vi "CRYFlatten User Equation Cluster.vi"(11 "user equation cluster":T1 {"Results axis" items=["x", "y", "z"]; "Input axis" items=["x", "y", "z"]; "Custom unit results array"."dB ref" format="%.2f"; "Custom unit input array"."dB ref" format="%.2f"}) -> (3 "Flatten String":string)   [LabVIEW 2013]
uses:
  Typedef Control/CRYUser Equation Cluster.ctl
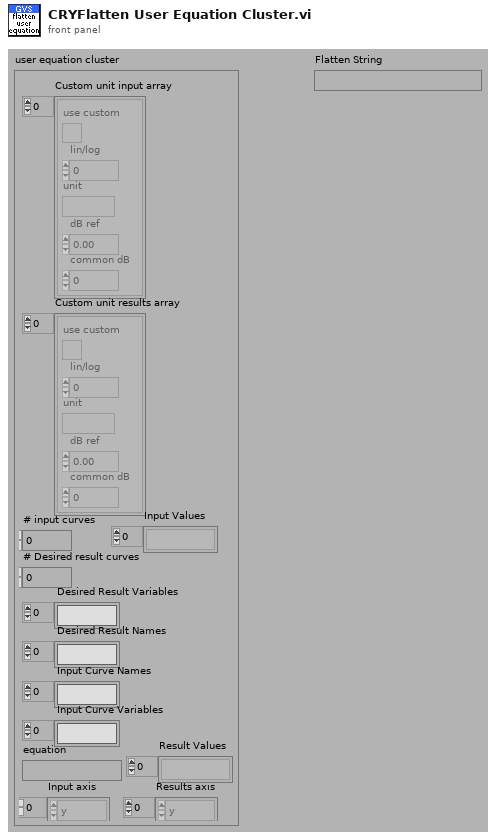
[diagram p1: front panel]
types:
  T1 = typedef "CRYUser Equation Cluster.ctl" = cluster{"Custom unit input array":cluster{"use custom":bool, "lin/log":u16, "unit":string, "dB ref":dbl, "common dB":u16}[], "Custom unit results array ":cluster{"use custom":bool, "lin/log":u16, "unit":string, "dB ref":dbl, "common dB":u16}[], "Desired Result Variables":string[], "Desired Result Names":string[], "Input Curve Names":string[], "Input Curve Variables":string[], "equation":string, "Input axis":u16[], "Results axis":u16[], "# input curves":i32, "# Desired result curves ":i32, "Input Values":string[], "Result Values":string[]}
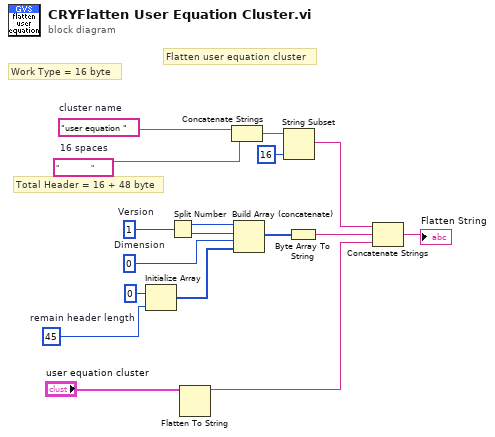
[diagram p0: block diagram]
diagram:
  w2 = "                "  # 16 spaces
  w3 = "user equation "  # cluster name
  w8 = u16 1  # Version
  w11 = u8 0  # Dimension
  w7 = 45  # remain header length
  # "Flatten user equation cluster"
  # "Work Type = 16 byte"
  # "Total Header = 16 + 48 byte"
  n1 = Initialize Array(u8 0 ("element"), w7) -> (w13:u8[])
  n2 = Split Number(x=w8) -> (hi(x)=w9:u8, lo(x)=w10:u8)
  n3 = Flatten To String(anything="user equation cluster") -> (data string=w14:string)  [unwired: 1 in, 4 out]
  n4 = Concatenate Strings(w3, w2) -> (w4:string)
  n5 = Build Array (concatenate)(w9, w10, w11, w13) -> (w12:u8[])
  n6 = String Subset(string=w4, length (rest)=16 ("length (rest)")) -> (substring=w16:string)  [unwired: 1 out]
  n7 = Byte Array To String(unsigned byte array=w12) -> (string=w15:string)
  n8 = Concatenate Strings(w16, w15, w14) -> (→"Flatten String":string)
